vi "Unit Vector (DBL).vi"(9 "user defined norm":dbl=-1.0, 10 "norm type":T1=2 items=["1-norm"=1, "2-norm"=2, "Inf-norm"=3, "-Inf-norm"=4, "User Defined"=5], 11 "Input Vector":dbl[](array[numeric]) format="%0.2f") -> (0 "error":i32, 2 "norm":dbl format="%0.2f", 3 "Unit Vector":dbl[](array[numeric]) format="%0.2f")   [LabVIEW 2017, in "NI_AALBase.lvlib"]
doc: "Finds the <B>norm</B> of the <B>Input Vector</B> and obtains its corresponding <B>Unit Vector</B> by normalizing the original <B>Input Vector</B> with its <B>norm</B>."
uses:
  NI_AALBase.lvlib
  Vector Norm Type.ctl
  <resource>/lvanlys.dll
  NI_AALPro.lvlib
panel:
  # "Unit Vector"
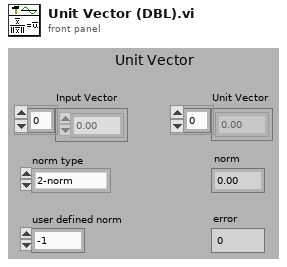
[diagram p1: front panel]
types:
  T1 = typedef "NI_AALPro.lvlib/Vector Norm Type.ctl" = u16
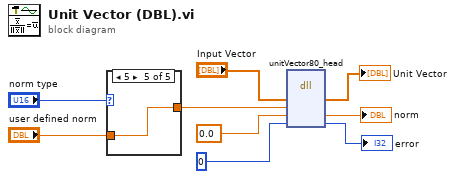
[diagram p0: block diagram]
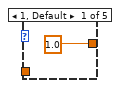
[diagram p2: hidden frame]
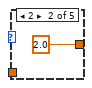
[diagram p3: hidden frame]
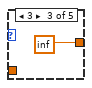
[diagram p4: hidden frame]
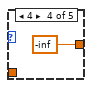
[diagram p5: hidden frame]
diagram:
  n1 = case shown="5" "norm type" {
    tunnel: [1.0 2.0 inf -inf w14] -> w1
    tunnel: "user defined norm" -> [_ _ _ _ w14]
    frame 1, Default {
    }
    frame 2 {
    }
    frame 3 {
    }
    frame 4 {
    }
    frame 5 {
    }
  }
  n2 = dll-call lib="C:/Program Files (x86)/National Instruments/LabVIEW 2017/resource/lvanlys.*" fn="unitVector80_head"("xH"="Input Vector", "p"=w1, "norm"=0.0, "dsperr"=0) -> ("xH"=→"Unit Vector":dbl[], "norm"=→"norm":dbl, "dsperr"=→"error":i32)  [unwired: 5 in, 2 out]
